vi "Roller Lift Control.vi"(8 "error in (no error)":errorcluster, 10 "Down":bool=TRUE, 11 "Up":bool=TRUE) -> (0 "error out":errorcluster, 3 "Roller Up/Down":T1)   [LabVIEW 2013]
uses:
  <vilib>/Rock Robotics/WPI/Solenoid/WPI_SolenoidValue.ctl
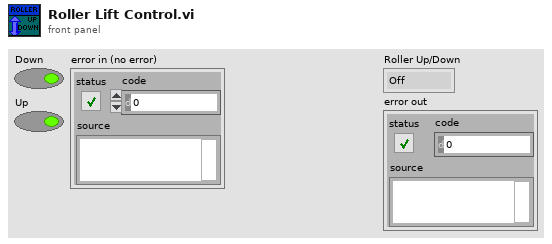
[diagram p1: front panel]
types:
  T1 = typedef "WPI_SolenoidValue.ctl" = enum16{"Off", "On", "Forward", "Reverse"}
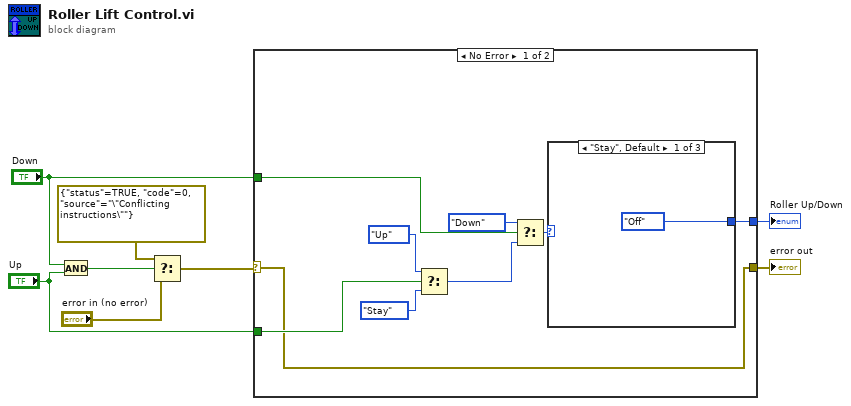
[diagram p0: block diagram]
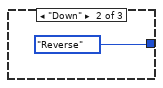
[diagram p2: hidden frame]
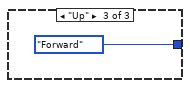
[diagram p3: hidden frame]
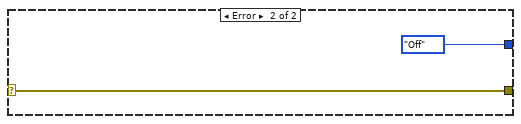
[diagram p4: hidden frame]
diagram:
  n1 = And(x="Down", y="Up") -> (x .and. y?=w6:bool)
  n2 = Select(t=errorcluster {"status"=TRUE, "code"=0, "source"="\"Conflicting instructions\""}, s=w6, f="error in (no error)") -> (s? t:f=w4:errorcluster)
  n3 = case shown="No Error" w4 {
    selector: w4 -> [w10 w22]
    tunnel: "Up" -> [w14 _]
    tunnel: "Down" -> [w11 _]
    tunnel: [w10 w22] -> w1
    tunnel: [w9 WPI_SolenoidValue."Off" ("Value")] -> w2
    frame No Error {
      n4 = Select(t=enum16{"Stay", "Down", "Up"}."Up", s=w14, f=enum16{"Stay", "Down", "Up"}."Stay") -> (s? t:f=w12:enum16{"Stay", "Down", "Up"})
      n5 = Select(t=enum16{"Stay", "Down", "Up"}."Down", s=w11, f=w12) -> (s? t:f=w15:enum16{"Stay", "Down", "Up"})
      n6 = case shown="\"Stay\", Default" w15 {
        tunnel: [WPI_SolenoidValue."Off" ("Value") WPI_SolenoidValue."Reverse" ("Value") WPI_SolenoidValue."Forward" ("Value")] -> w9
        frame "Stay", Default {
        }
        frame "Down" {
        }
        frame "Up" {
        }
      }
    }
    frame Error {
    }
  }
  "Roller Up/Down" <- w2
  "error out" <- w1
